vi "Host_PulseHistogram.vi"() -> ()   [LabVIEW 2012]
uses:
  <vilib>/FPGAPlugInAG/PXIe-7962R/niLvFpga_Open_PXIe-7962R.vi
  <vilib>/rvi/interface/common/dynamic/niFpgaDynamicAddResources.vi
  <vilib>/Utility/error.llb/Error Cluster From Error Code.vi
  <vilib>/rvi/errors/niLvFpgaAdjustHostInterfaceError.vi
  <vilib>/FPGAPlugInAG/Dynamic/niLvFpga_Close_Dynamic.vi
  <vilib>/rvi/interface/nirviOpenFPGA/nirviOpenFPGA.xnode
  FPGA Bitfiles/PulseHistogram_PXIe-7962R.lvbitx
  <vilib>/rvi/interface/nirviReadWriteControl/nirviReadWriteControl.xnode
  <vilib>/rvi/interface/nirviMethod/nirviMethod.xnode
  <vilib>/rvi/interface/nirviCloseFPGA/nirviCloseFPGA.xnode
  <vilib>/rvi/interface/Simulation/niFpgaSimulationCallBeginRW.vi
  <vilib>/rvi/errors/niLvFpgaMergeErrorWithErrorCode.vi
  NiFpgaLv.dll
  <vilib>/FPGAPlugInAG/Dynamic/niLvFpga_ReadFifo_Dynamic.vi
  <vilib>/FPGAPlugInAG/Dynamic/niLvFpga_ConfigureFifo_Dynamic.vi
panel:
  out "Relative probe pulse period histogram A1":T1(graph)
  in  "Demultiplex":bool
  out "Probe pulse histogram A2":T1(graph)
  out "Total probe pulse count A2":u64
  out "Relative probe pulse period histogram A2":T1(graph)
  out "Loop counter":i32
  out "Waveform Graph":waveform(i16)[](graph)
  out "Interloop FIFO timed out":bool
  out "Acq FIFO overflow":bool
  out "Interloop FIFO overflow":bool
  out "Probe pulses per second A1":dbl
  out "Total probe pulse count A1":u64
  out "Probe pulse histogram A1":T1(graph)
  out "Reference pulse frequency":dbl format="%#_5p"
  out "Total sample count":u64
  out "Total reference pulse count":u64
  out "Elements Remaining":u32
  out "Reference pulse length histogram":T1(graph)
  out "Reference pulse period histogram":T1(graph)
  out "Sampling frequency":dbl format="%#_6p"
  out "Sampling interval":dbl format="%#_6p"
  in  "Onboard clock frequency":dbl=500000000.0 format="%#_6p"
  in  "Quit":bool
  # "Set before start!"
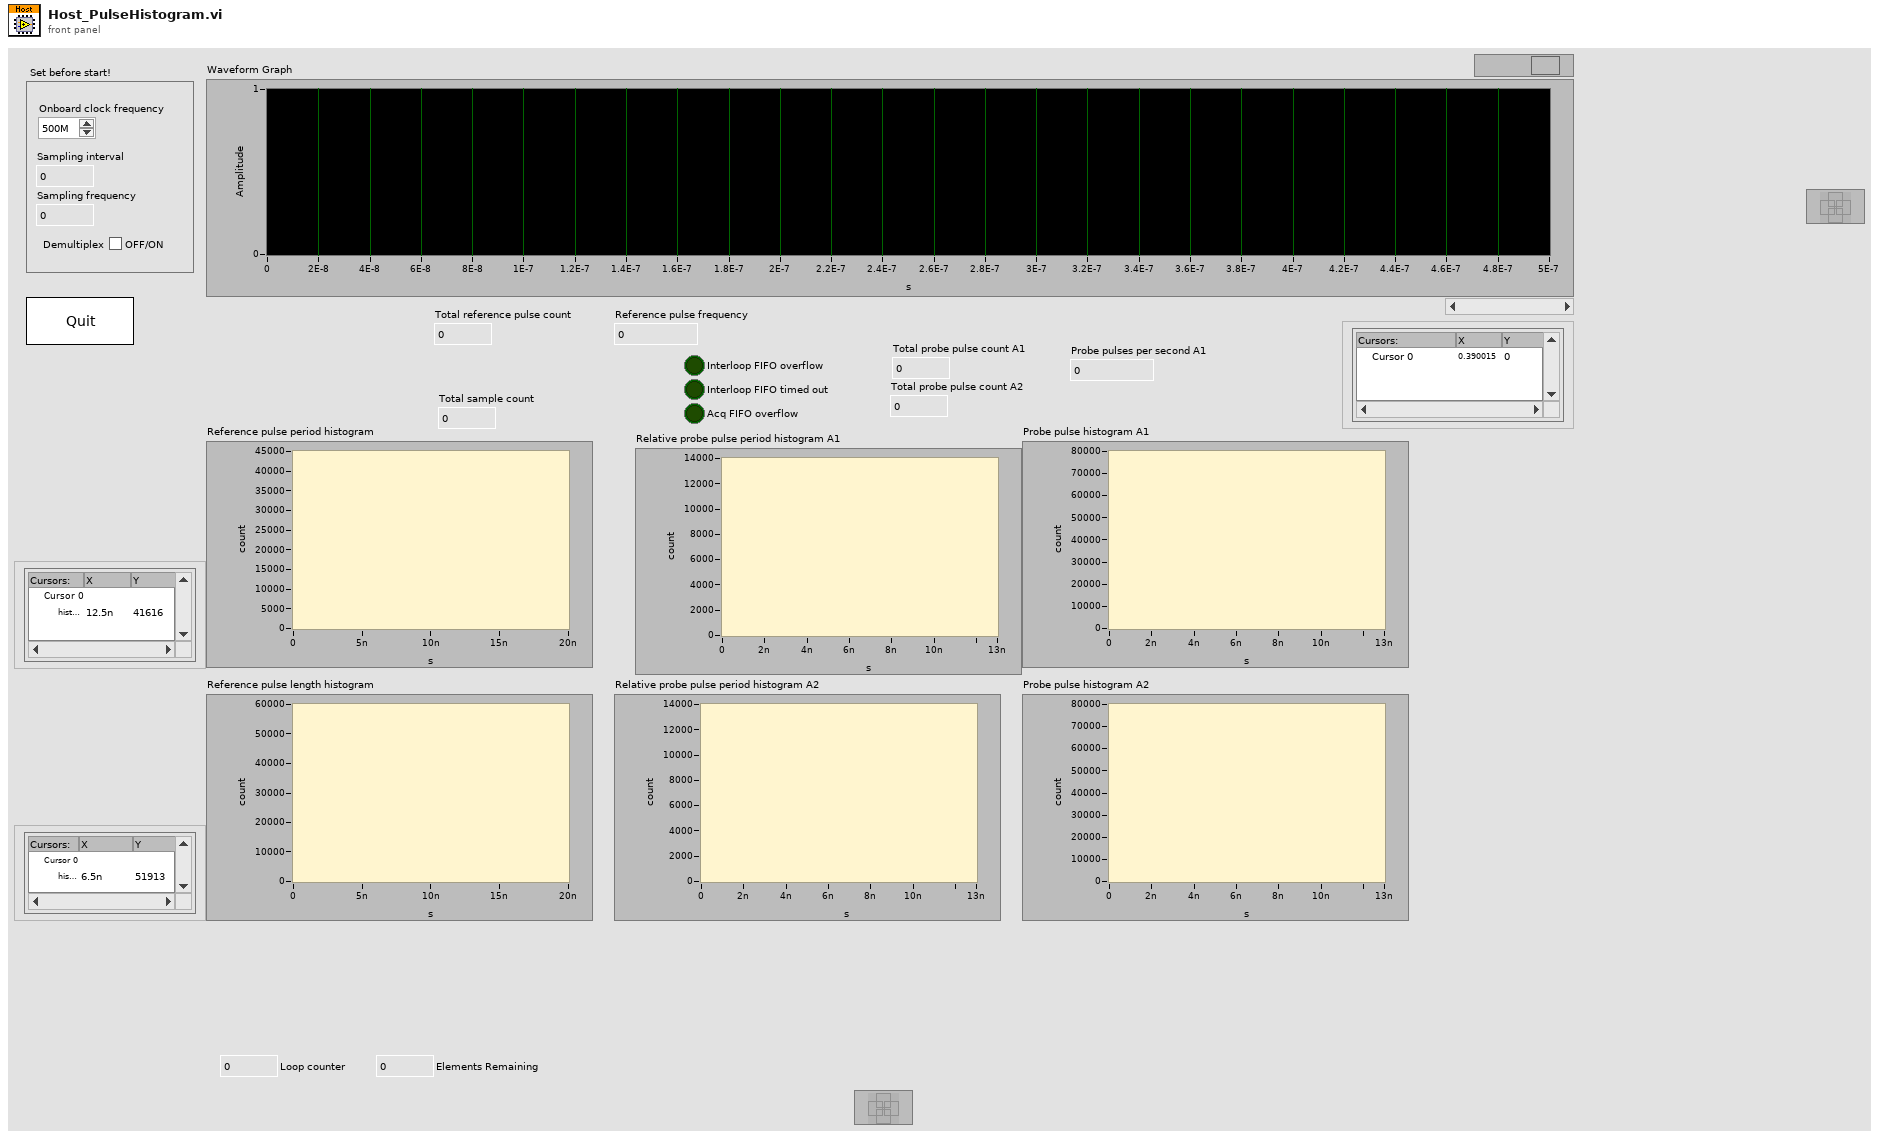
[diagram p1: front panel]
types:
  T1 = cluster{"X Values":dbl[], "Histogram: h(x)":i32[]}
  T2 = enum8{"Enabled", "Disabled", "Disabled and Grayed Out"}
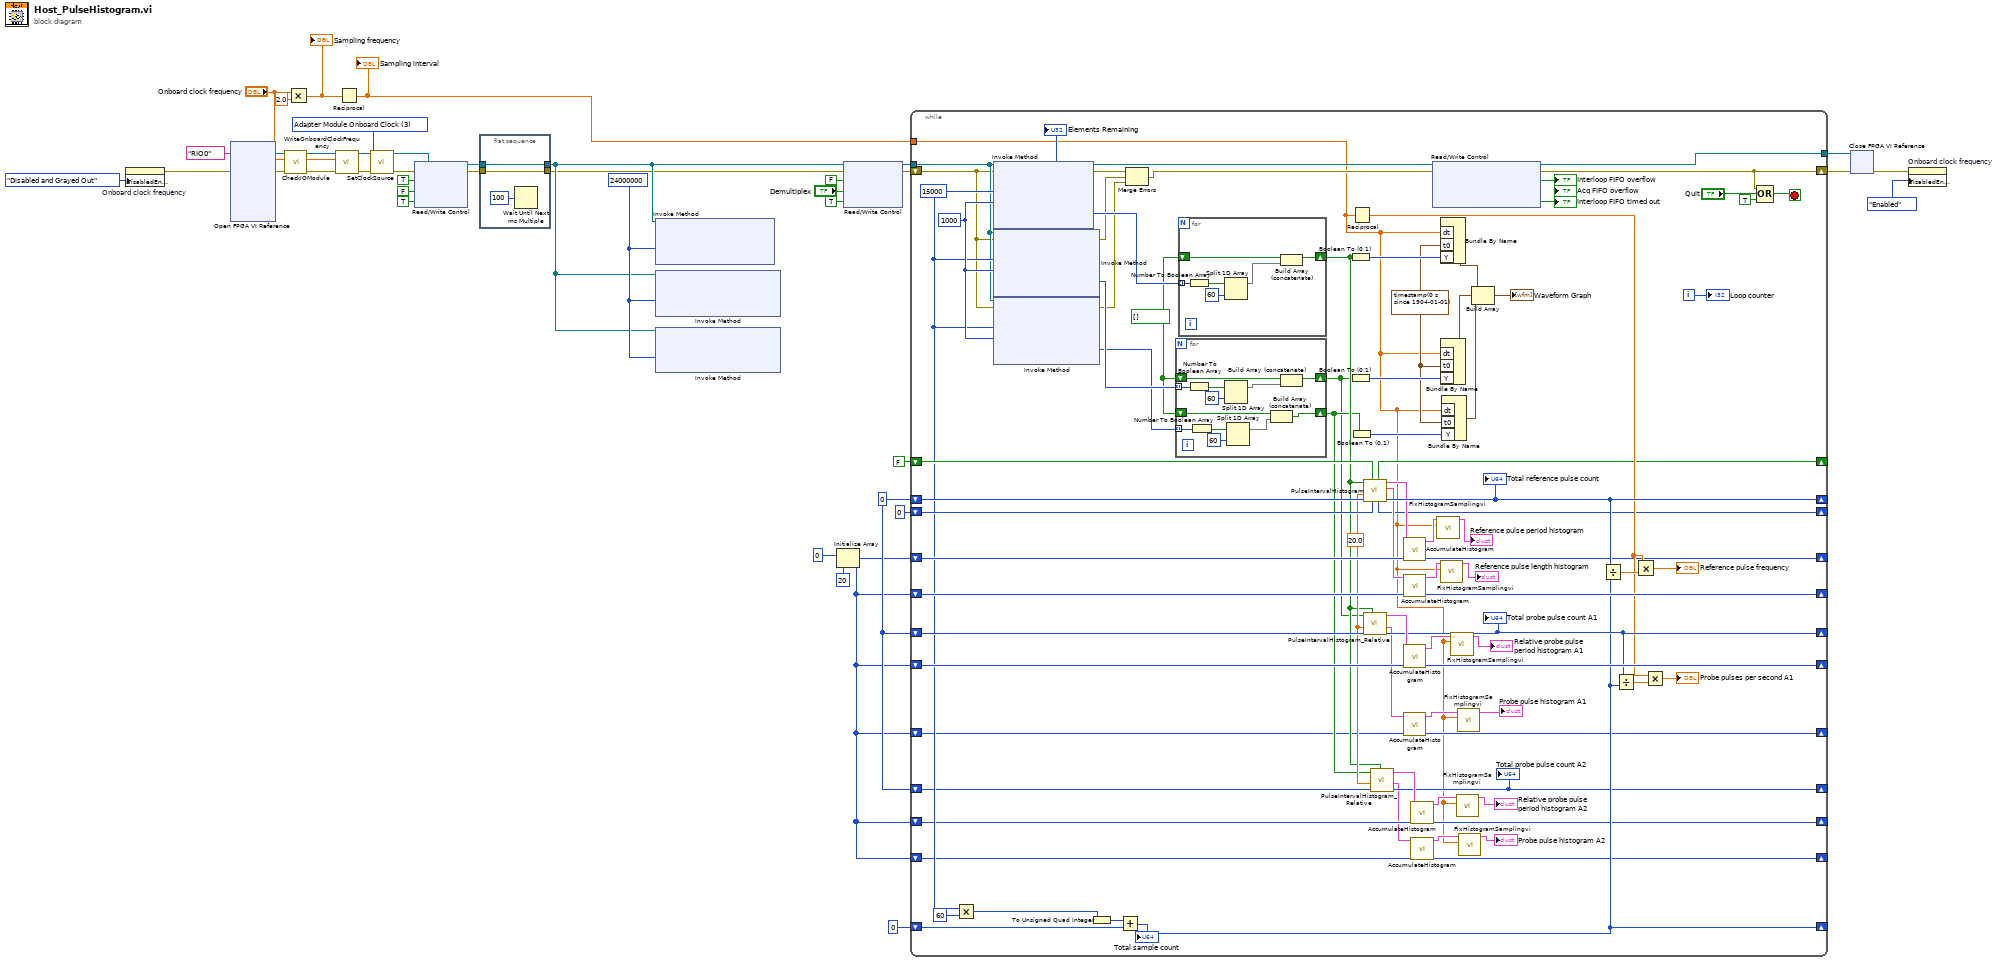
[diagram p0: block diagram]
diagram:
  w7 = u32 24000000 ("Samples to acquire")
  w4 = u64 0 ("Pulse count out")
  w40 = u8 3 items=["Tristate"=0, "Sync Clock (PXIe only)"=2, "Adapter Module Onboard Clock"=3, "Strobe from Crosspoint Switch"=4, "Strobe Bypass"=5] ("Clock Source")
  n1 = property on="Onboard clock frequency" class="DigNum (strict)"("DisabledEnum"=T2."Disabled and Grayed Out" ("Disabled")) -> (error out=w24:errorcluster)  [unwired: 2 in, 1 out]
  n2 = xnode "Open FPGA VI Reference"("error in"=w24, "resource name"=tag "RIO0") -> ("FPGA VI Reference Out"=w9:refnum<k20>, "error out"=w8:errorcluster)
  n3 = call "CheckIOModule.vi"("error in (no error)"=w8, "FPGA VI Reference In"=w9) -> ("error out"=w34:errorcluster, "FPGA VI Reference Out"=w33:refnum<k20>)  [unwired: 8 in]
  n4 = Multiply(x="Onboard clock frequency", y=2.0) -> (x*y=w28:dbl)
  "Sampling frequency" <- w28
  n5 = call "WriteOnboardClockFrequency.vi"("error in (no error)"=w34, "Onboard clock frequency"="Onboard clock frequency", "FPGA VI Reference In"=w33) -> ("error out"=w32:errorcluster, "FPGA VI Reference Out"=w31:refnum<k20>)  [unwired: 7 in]
  n6 = Reciprocal(x=w28) -> (1/x=w27:dbl)
  "Sampling interval" <- w27
  n7 = call "SetClockSource.vi"("error in (no error)"=w32, "Clock Source"=w40, "FPGA VI Reference In"=w31) -> ("error out"=w38:errorcluster, "FPGA VI Reference Out"=w39:refnum<k20>)  [unwired: 7 in]
  n8 = xnode "Read/Write Control"("FPGA VI Reference In"=w39, "error in"=w38, "Commit"=TRUE, "Acq_Reset"=FALSE, "Acq_Reset"=TRUE) -> ("FPGA VI Reference Out"=w16:refnum<k20>, "error out"=w15:errorcluster)
  n9 = flat-sequence {
    tunnel: w16 -> [w41]
    tunnel: w15 -> [w42]
    tunnel: [w42] -> w5
    tunnel: [w41] -> w6
    frame #0 {
      n10 = Wait Until Next ms Multiple(millisecond multiple=u32 100) -> ()  [unwired: 1 out]
    }
  }
  n11 = xnode "Invoke Method"("FPGA VI Reference In"=w6, "Requested Depth"=w7) -> ()  [unwired: 1 in, 3 out]
  n12 = xnode "Invoke Method"("FPGA VI Reference In"=w6, "Requested Depth"=w7) -> ()  [unwired: 1 in, 3 out]
  n13 = xnode "Invoke Method"("FPGA VI Reference In"=w6, "Requested Depth"=w7) -> ()  [unwired: 1 in, 3 out]
  n14 = Initialize Array(0, 20 ("dimension size")) -> (w3:i32[])
  n15 = xnode "Read/Write Control"("FPGA VI Reference In"=w6, "error in"=w5, "Acq_Reset"=FALSE, "Demultiplex"="Demultiplex", "Acquiring"=TRUE) -> ("FPGA VI Reference Out"=w13:refnum<k20>, "error out"=w14:errorcluster)
  n16 = while {
    tunnel: w13 -> [w83]
    tunnel: w27 -> [w48]
    shift-right: [w91] -> w26
    shift-left: w14 -> [w82]
    tunnel: [w101] -> w25
    shift-right: [w93] -> _
    shift-left: w3 -> [w128]
    shift-right: [w127] -> _
    shift-left: w3 -> [w126]
    shift-right: [w125] -> _
    shift-left: w4 -> [w124]
    shift-right: [w108] -> _
    shift-left: u64 0 ("Pulse count out") -> [w123]
    shift-right: [w109] -> _
    shift-left: w4 -> [w113]
    shift-right: [w111] -> _
    shift-left: w3 -> [w110]
    shift-right: [w97] -> _
    shift-left: FALSE ("Last reference value out") -> [w96]
    shift-right: [w95] -> _
    shift-left: 0 ("Last rising flank out") -> [w94]
    shift-right: [w67] -> _
    shift-left: w4 -> [w66]
    shift-right: [w65] -> _
    shift-left: w3 -> [w63]
    shift-right: [w64] -> _
    shift-left: w3 -> [w62]
    shift-right: [w51] -> _
    shift-left: w3 -> [w52]
    i -> [w77]
    stop <- w92 stop-if-true
    w70 = 20.0 ("No of SI bins")
    w73 = timestamp(0 s since 1904-01-01) ("t0")
    w75 = bool[] []
    w87 = u32 15000 ("Number of Elements")
    w88 = 1000 ("Timeout (ms)")
    n17 = Multiply(x=w87, y=u32 60) -> (x*y=w115:u32)
    n18 = xnode "Invoke Method"("FPGA VI Reference In"=w83, "error in"=w82, "Number of Elements"=w87, "Timeout (ms)"=w88) -> ("FPGA VI Reference Out"=w89:refnum<k20>, "error out"=w81:errorcluster, "Data"=w86:u64[], "Elements Remaining"=→"Elements Remaining":u32)
    n19 = xnode "Invoke Method"("FPGA VI Reference In"=w83, "error in"=w82, "Number of Elements"=w87, "Timeout (ms)"=w88) -> ("error out"=w79:errorcluster, "Data"=w85:u64[])  [unwired: 2 out]
    n20 = xnode "Invoke Method"("FPGA VI Reference In"=w83, "error in"=w82, "Number of Elements"=w87, "Timeout (ms)"=w88) -> ("error out"=w78:errorcluster, "Data"=w84:u64[])  [unwired: 2 out]
    n21 = To Unsigned Quad Integer(1:w115) -> (0:w114:u64)
    n22 = Add(x=w114, y=w123) -> (x+y=w108:u64)
    "Total sample count" <- w108
    n23 = Merge Errors(w81, w79, w78) -> (w80:errorcluster)
    n24 = for {
      shift-right: [w138] -> w45
      shift-left: w75 -> [w137]
      tunnel: w85 -> [w135] mode=indexing
      tunnel: w84 -> [w132] mode=indexing
      shift-right: [w130] -> w68
      shift-left: w75 -> [w131]
      n25 = Number To Boolean Array(number=w135) -> (Boolean array=w140:bool[])
      n26 = Number To Boolean Array(number=w132) -> (Boolean array=w134:bool[])
      n27 = Split 1D Array(array=w140, index=60) -> (first subarray=w136:bool[])  [unwired: 1 out]
      n28 = Split 1D Array(array=w134, index=60) -> (first subarray=w129:bool[])  [unwired: 1 out]
      n29 = Build Array (concatenate)(w131, w129) -> (w130:bool[])
      n30 = Build Array (concatenate)(w137, w136) -> (w138:bool[])
    }
    n31 = for {
      shift-right: [w144] -> w69
      shift-left: w75 -> [w143]
      tunnel: w86 -> [w141] mode=indexing
      n32 = Number To Boolean Array(number=w141) -> (Boolean array=w146:bool[])
      n33 = Split 1D Array(array=w146, index=60) -> (first subarray=w142:bool[])  [unwired: 1 out]
      n34 = Build Array (concatenate)(w143, w142) -> (w144:bool[])
    }
    n35 = Boolean To (0,1)(Boolean=w69) -> (0, 1=w122:i16[])
    n36 = Boolean To (0,1)(Boolean=w45) -> (0, 1=w116:i16[])
    n37 = Reciprocal(x=w48) -> (1/x=w106:dbl)
    n38 = Boolean To (0,1)(Boolean=w68) -> (0, 1=w74:i16[])
    n39 = call "PulseIntervalHistogram.vi"("Last rising flank in"=w94, "Last reference value in"=w96, "Pulse count in"=w124, "No of SI bins"=w70, "Binary array probe"=w69) -> ("Pulse count out"=w125:u64, "Pulse length histogram"=w120:T1, "Pulse period histogram"=w121:T1, "Last rising flank out"=w95:i32, "Last reference value out"=w97:bool)  [unwired: 1 in, 1 out]
    "Total reference pulse count" <- w125
    n40 = call "PulseIntervalHistogram_Relative.vi"("Binary array reference"=w69, "Pulse count in"=w113, "No of SI bins"=w70, "Binary array probe"=w45) -> ("Pulse count out"=w109:u64, "Pulse histogram"=w50:T1, "Pulse period histogram"=w112:T1)  [unwired: 4 in, 1 out]
    "Total probe pulse count A1" <- w109
    n41 = call "PulseIntervalHistogram_Relative.vi"("Binary array reference"=w69, "Pulse count in"=w66, "No of SI bins"=w70, "Binary array probe"=w68) -> ("Pulse count out"=w67:u64, "Pulse histogram"=w46:T1, "Pulse period histogram"=w71:T1)  [unwired: 4 in, 1 out]
    "Total probe pulse count A2" <- w67
    n42 = call "AccumulateHistogram.vi"("Array in"=w128, "Histogram graph in"=w121) -> ("Array out"=w93:i32[], "Histogram graph out"=w61:T1)  [unwired: 8 in]
    n43 = call "AccumulateHistogram.vi"("Array in"=w126, "Histogram graph in"=w120) -> ("Array out"=w127:i32[], "Histogram graph out"=w59:T1)  [unwired: 8 in]
    n44 = call "AccumulateHistogram.vi"("Array in"=w110, "Histogram graph in"=w112) -> ("Array out"=w111:i32[], "Histogram graph out"=w57:T1)  [unwired: 8 in]
    n45 = call "AccumulateHistogram.vi"("Array in"=w52, "Histogram graph in"=w50) -> ("Array out"=w51:i32[], "Histogram graph out"=w49:T1)  [unwired: 8 in]
    n46 = call "AccumulateHistogram.vi"("Array in"=w63, "Histogram graph in"=w71) -> ("Array out"=w65:i32[], "Histogram graph out"=w56:T1)  [unwired: 8 in]
    n47 = call "AccumulateHistogram.vi"("Array in"=w62, "Histogram graph in"=w46) -> ("Array out"=w64:i32[], "Histogram graph out"=w54:T1)  [unwired: 8 in]
    n48 = xnode "Read/Write Control"("FPGA VI Reference In"=w89, "error in"=w80) -> ("FPGA VI Reference Out"=w101:refnum<k20>, "error out"=w91:errorcluster, "Interloop FIFO overflow"=→"Interloop FIFO overflow":bool, "Interloop FIFO timed out"=→"Interloop FIFO timed out":bool)  [unwired: 1 out]
    n49 = call "FixHistogramSamplingvi.vi"("Sampling Interval"=w48, "Histogram in"=w61) -> ("Histogram out"=→"Reference pulse period histogram":T1)  [unwired: 9 in]
    n50 = Bundle By Name("dt"=w48, "t0"=w73, "Y"=w122) -> (w100:waveform(i16))  [unwired: 1 in]
    n51 = Bundle By Name("dt"=w48, "t0"=w73, "Y"=w116) -> (w99:waveform(i16))  [unwired: 1 in]
    n52 = call "FixHistogramSamplingvi.vi"("Sampling Interval"=w48, "Histogram in"=w59) -> ("Histogram out"=→"Reference pulse length histogram":T1)  [unwired: 9 in]
    n53 = Bundle By Name("dt"=w48, "t0"=w73, "Y"=w74) -> (w72:waveform(i16))  [unwired: 1 in]
    n54 = call "FixHistogramSamplingvi.vi"("Sampling Interval"=w48, "Histogram in"=w57) -> ("Histogram out"=→"Relative probe pulse period histogram A1":T1)  [unwired: 9 in]
    n55 = call "FixHistogramSamplingvi.vi"("Sampling Interval"=w48, "Histogram in"=w56) -> ("Histogram out"=→"Relative probe pulse period histogram A2":T1)  [unwired: 9 in]
    n56 = call "FixHistogramSamplingvi.vi"("Sampling Interval"=w48, "Histogram in"=w49) -> ("Histogram out"=→"Probe pulse histogram A1":T1)  [unwired: 9 in]
    n57 = call "FixHistogramSamplingvi.vi"("Sampling Interval"=w48, "Histogram in"=w54) -> ("Histogram out"=→"Probe pulse histogram A2":T1)  [unwired: 9 in]
    n58 = Build Array(w100, w99, w72) -> (→"Waveform Graph":waveform(i16)[])
    n59 = Divide(x=w125, y=w108) -> (x/y=w118:dbl)
    n60 = Divide(x=w109, y=w108) -> (x/y=w107:dbl)
    n61 = Multiply(x=w106, y=w118) -> (x*y=→"Reference pulse frequency":dbl)
    n62 = Multiply(x=w106, y=w107) -> (x*y=→"Probe pulses per second A1":dbl)
    n63 = Compound Arithmetic op=OR(w91, "Quit", TRUE ("value")) -> (w92:bool)
    "Loop counter" <- w77
  }
  n64 = xnode "Close FPGA VI Reference"("FPGA VI Reference In"=w25, "error in"=w26) -> ("error out"=w22:errorcluster)
  n65 = property on="Onboard clock frequency" class="DigNum (strict)"(error in=w22, "DisabledEnum"=T2."Enabled" ("Disabled")) -> ()  [unwired: 1 in, 2 out]
